vi "sub_time_to_string.vi"(8 "error in (no error)":errorcluster, 11 "timestamp":timestamp) -> (0 "error out":errorcluster, 3 "time":string)   [LabVIEW 2013, in "daqio minimal.lvlib"]
doc: "This returns a string representation of a given timestamp. If no timestamp is given, it will return the current system time."
uses:
  daqio minimal.lvlib
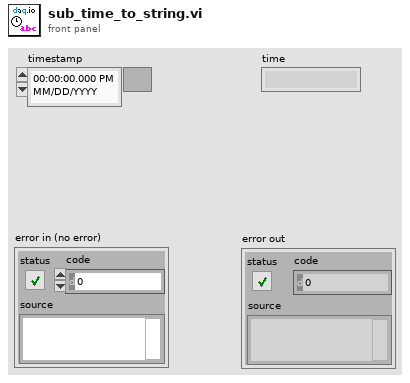
[diagram p1: front panel]
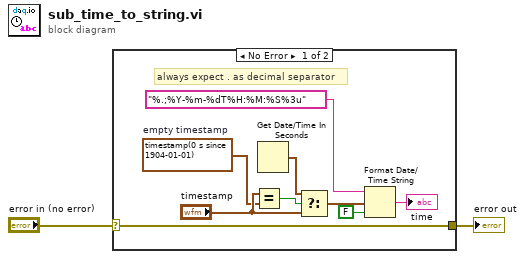
[diagram p0: block diagram]
diagram:
  n1 = case shown="No Error" "error in (no error)" {
    selector: "error in (no error)" -> [w3 w12]
    tunnel: [w3 w12] -> w1
    frame No Error {
      w8 = timestamp(0 s since 1904-01-01)  # empty timestamp
      # "always expect . as decimal separator"
      n2 = Equal?(x="timestamp", y=w8) -> (x = y?=w9:bool)
      n3 = Get Date/Time In Seconds() -> (seconds since 1Jan1904=w10:timestamp)
      n4 = Select(t=w10, s=w9, f="timestamp") -> (s? t:f=w5:timestamp)
      n5 = Format Date/Time String(time format string (%c)="%.;%Y-%m-%dT%H:%M:%S%3u", seconds (now)=w5, UTC format=FALSE) -> (date/time string=→"time":string)
    }
    frame Error {
    }
  }
  "error out" <- w1
